vi "sub_DTMF_Encoder.vi"(8 "Dial Tone":bool, 11 "digits":u8[](array[numeric])) -> (3 "signal":dbl[](array[numeric]))   [LabVIEW 2011]
uses:
  <vilib>/imath/engines/lvmath/Plug In/_Char/NIMS_CH_character datatype.ctl
  <vilib>/imath/engines/lvmath2/RunTimeEngine/ErrorHandling/NIMS_Finalize Error.vi
  <vilib>/imath/engines/lvmath2/RunTimeEngine/Managers/WorkSpace/UID Generator.vi
  <vilib>/imath/engines/lvmath2/RunTimeEngine/BuiltInFunctions/length/NIMS_length(GV).vi
  <instcachedir>/0/NIMS_length(GV)_08A3D13377FD4E4B96F5795FBF3698FA.lvgen/NIMS_length(GV)_08A3D13377FD4E4B96F5795FBF3698FA_003.vi
  <vilib>/imath/engines/lvmath2/RunTimeEngine/Managers/SymbolTable/Clear UID.vi
  <vilib>/imath/engines/lvmath2/RunTimeEngine/NodeEndStatement/NIMS_NodeEndStatement_Output.vi
  <instcachedir>/0/NIMS_NodeEndStatement_Output_53EC0D466D134D7ABD903AC30B43404B.lvgen/NIMS_NodeEndStatement_Output_53EC0D466D134D7ABD903AC30B43404B_005.vi
  <vilib>/imath/engines/lvmath2/RunTimeEngine/RangeToken/NIMS_Range.vi
  <instcachedir>/0/NIMS_Range_0B7635FB69F84E19AA68E7FF959DF37C.lvgen/NIMS_Range_0B7635FB69F84E19AA68E7FF959DF37C_001.vi
  <vilib>/imath/engines/lvmath2/RunTimeEngine/ArithmeticOperatorToken/NIMS_ArithmeticOperator_plus.vi
  <instcachedir>/0/NIMS_ArithmeticOperator_plus_1E95F7DAB906458CBECCADBE8E6FD739.lvgen/NIMS_ArithmeticOperator_plus_1E95F7DAB906458CBECCADBE8E6FD739_004.vi
  <vilib>/imath/engines/lvmath2/RunTimeEngine/ErrorHandling/NIMS_Create Error From Enums.vi
  <vilib>/imath/engines/lvmath2/RunTimeEngine/RangeToken/NIMS_Range_R2 - Integer.vi
  <instcachedir>/0/NIMS_Range_R2 - Integer_8B99B1FAA0BB43C693F13B8216F464EC.lvgen/NIMS_Range_R2 - Integer_8B99B1FAA0BB43C693F13B8216F464EC_000.vi
  <vilib>/imath/engines/lvmath2/RunTimeEngine/CommandStatement/MC_CommandStatement_break.vi
  <vilib>/imath/engines/lvmath2/RunTimeEngine/BuiltInFunctions/rand/NIMS_rand().vi
  <vilib>/imath/engines/lvmath2/RunTimeEngine/BuiltInFunctions/round/NIMS_round(DBL-S).vi
  <vilib>/imath/engines/lvmath2/RunTimeEngine/ErrorHandling/NIMS_Error From Error Code.vi
  <vilib>/imath/engines/lvmath2/RunTimeEngine/BuiltInFunctions/zeros/NIMS_V=zeros(I32,I32).vi
  <vilib>/imath/engines/lvmath2/RunTimeEngine/RowToken/NIMS_RowToken_M_SorRV.vi
  <instcachedir>/0/NIMS_RowToken_M_SorRV_7D706DDE498144F993BC9D4030E937C1.lvgen/NIMS_RowToken_M_SorRV_7D706DDE498144F993BC9D4030E937C1_000.vi
  <vilib>/imath/engines/lvmath2/RunTimeEngine/VariableToken/Read/NIMS_Get Elements - RV(_) - Check.vi
  <instcachedir>/0/NIMS_Get Elements - RV(_) - Check_B511B9D8E05044FE80F9F088FE24B20C.lvgen/NIMS_Get Elements - RV(_) - Check_B511B9D8E05044FE80F9F088FE24B20C_003.vi
  <vilib>/imathl/engines/lvmath/Functions/Error Handling/Create Error.vi
  <vilib>/imath/engines/lvmath2/RunTimeEngine/RunTimeType/NIMS_RunTimeType_From StrictType (excl LVString).vi
  <instcachedir>/0/NIMS_RunTimeType_From StrictType (excl LVString)_46AE8B54A11948F0BCCEB8091EE7AA4C.lvgen/NIMS_RunTimeType_From StrictType (excl LVString)_46AE8B54A11948F0BCCEB8091EE7AA4C_001.vi
  <vilib>/imath/engines/lvmath2/RunTimeEngine/LocalVariableDefStatement/MC_LocalVariableDefStatement_Display.vi
  <vilib>/imath/engines/lvmath2/RunTimeEngine/BuiltInFunctions/quit/NIMS_quit.vi
  <vilib>/imath/engines/lvmath2/RunTimeEngine/VariableToken/Read/NIMS_Get Elements - V(S).vi
  <instcachedir>/0/NIMS_Get Elements - V(S)_C99A26467DB24FA3A79619D034B25FD8.lvgen/NIMS_Get Elements - V(S)_C99A26467DB24FA3A79619D034B25FD8_000.vi
  <vilib>/imath/engines/lvmath2/RunTimeEngine/VariableToken/NIMS_VariableToken_CondDefined.vi
  <instcachedir>/0/NIMS_VariableToken_CondDefined_D30D2F4D3CE04567BC79CC35D27951F7.lvgen/NIMS_VariableToken_CondDefined_D30D2F4D3CE04567BC79CC35D27951F7_004.vi
  <vilib>/imath/engines/lvmath2/RunTimeEngine/BuiltInFunctions/abs/NIMS_abs(signed).vi
  <instcachedir>/0/NIMS_abs(signed)_C4FCB8E6058B49B797C7C8D53CA5F6EC.lvgen/NIMS_abs(signed)_C4FCB8E6058B49B797C7C8D53CA5F6EC_001.vi
  <vilib>/imath/engines/lvmath2/RunTimeEngine/BuiltInFunctions/max/1 input/NIMS_max(RV).vi
  <instcachedir>/0/NIMS_max(RV)_237633DB1D604D5BA7001287DF3C7957.lvgen/NIMS_max(RV)_237633DB1D604D5BA7001287DF3C7957_000.vi
  <vilib>/imath/engines/lvmath2/RunTimeEngine/BuiltInFunctions/soundscaled/NIMS_soundscaled.vi
  <vilib>/imath/engines/lvmath2/RunTimeEngine/Managers/SymbolTable/NIMS_WorkSpace.lvlib
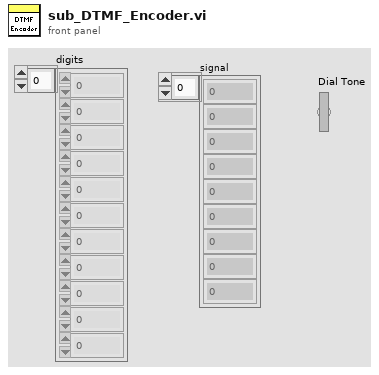
[diagram p1: front panel]
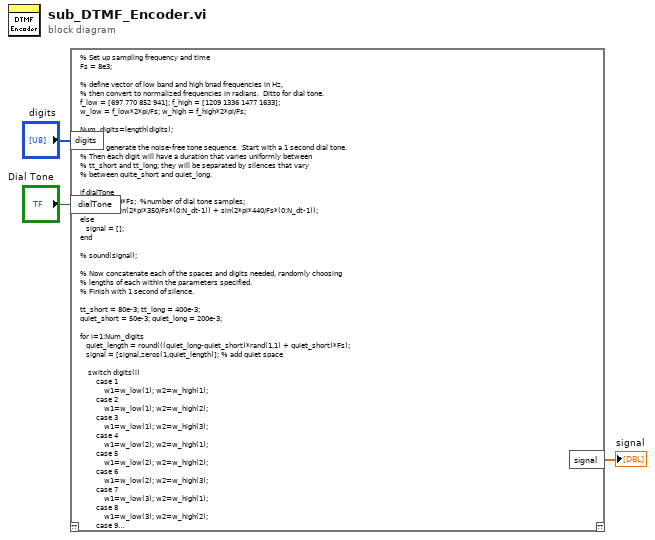
[diagram p0: block diagram]
diagram:
  n1 = mathscript code="% Set up sampling frequency and time\nFs = 8e3;\n\n% define vector of low band and high bnad frequencies in Hz,\n% then convert to normalized frequencies in radians.  Ditto for dial tone.\nf_low = [697 770 852 941]; f_high = [1209 1336 1477 1633];\nw_low = f_low*2*pi/Fs; w_high = f_high*2*pi/Fs;\n\nNum_digits=length(digits);\n\n% Now generate the noise-free tone sequence.  Start with a 1 second dial tone.\n% Then each digit will have a duration that varies uniformly between\n% tt_short and tt_long; they will be separated by silences that vary\n% between quite_short and quiet_long.\n\nif dialTone\n   N_dt = 1.0*Fs;  %number of dial tone samples;\n   signal = sin(2*pi*350/Fs*(0:N_dt-1)) + sin(2*pi*440/Fs*(0:N_dt-1));\nelse\n   signal = [];\nend\n\n% sound(signal);\n\n% Now concatenate each of the spaces and digits needed, randomly choosing\n% lengths of each within the parameters specified.\n% Finish with 1 second of silence.\n\ntt_short = 80e-3; tt_long = 400e-3;\nquiet_short = 50e-3; quiet_long = 200e-3;\n\nfor i=1:Num_digits\n   quiet_length = round(((quiet_long-quiet_short)*rand(1,1) + quiet_short)*Fs);\n   signal = [signal,zeros(1,quiet_length)]; % add quiet space\n    \n    switch digits(i)\n        case 1\n            w1=w_low(1); w2=w_high(1);\n        case 2\n            w1=w_low(1); w2=w_high(2);\n        case 3\n            w1=w_low(1); w2=w_high(3);\n        case 4\n            w1=w_low(2); w2=w_high(1);\n        case 5\n            w1=w_low(2); w2=w_high(2);\n        case 6\n            w1=w_low(2); w2=w_high(3);\n        case 7\n            w1=w_low(3); w2=w_high(1);\n        case 8\n            w1=w_low(3); w2=w_high(2);\n        case 9\n            w1=w_low(3); w2=w_high(3);\n        case 0\n            w1=w_low(4); w2=w_high(2);\n        otherwise\n            disp('Error: non-numeric touch tone input.')\n            exit\n    end\n\ttt_length = round(((tt_long-tt_short)*rand(1,1) + tt_short)*Fs);\n    n=0:tt_length-1;\n    tone = sin(w1*n) + sin(w2*n);\n    signal = [signal,tone];\nend\n\n% add one more second of quiet at the end\nsignal = [signal, zeros(1,Fs)];\n\n% Now for noise.  Power in a real sinusoid of amplitude A is A^2/2;\n% for sum of 2 non-harmonic sinusoids we will consider it to be\n% sum of their separate powers, so A^2.  In this M file, A=1, so\n% power of each touch tone pair is assumed to be 1.0.\n% Power of Gaussian noise is its variance, so we set variance to\n% get desired SNR and add zero mean Gaussian noise.\n\n% Scale to maximum amplitude of 1\n\nsignal = signal/max(abs(signal));\n\nsoundsc(signal, 8000)"("digits"="digits", "dialTone"="Dial Tone") -> ("signal"=→"signal":dbl[])  [unwired: 1 in, 1 out]
